vi "Test is a JKI State Machine.vi"(8 "error in (no error)":errorcluster) -> (0 "error out":errorcluster)   [LabVIEW 2013, in "TEST JKI State Machine API.lvlib"]
uses:
  TEST JKI State Machine API.lvlib
  <vilib>/addons/_JKI Toolkits/Caraya/classes/Test/Test.lvclass
  source/JKI SM/JKI SM.lvclass
  <vilib>/addons/_JKI Toolkits/Caraya/classes/Assert/Assert.lvclass
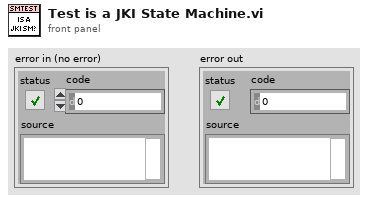
[diagram p1: front panel]
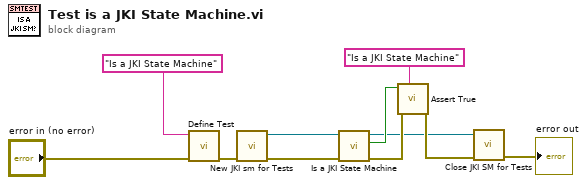
[diagram p0: block diagram]
diagram:
  n1 = call <vilib>:"Define Test.vi"("error in (no error)"="error in (no error)", "Label (VI Title)"="Is a JKI State Machine") -> ("error out"=w7:errorcluster)  [unwired: 9 in]
  n2 = call "New JKI sm for Tests.vi"("error in (no error)"=w7) -> ("error out"=w6:errorcluster, "JKI SM out"=w5:refnum<class "JKI SM.lvclass">)  [unwired: 9 in]
  n3 = call "Is a JKI State Machine.vi"("error in (no error)"=w6, "JKI SM in"=w5) -> ("error out"=w9:errorcluster, "Is a JKI State Machine"=w8:bool, "JKI SM out"=w1:refnum<class "JKI SM.lvclass">)  [unwired: 7 in]
  n4 = call <vilib>:"Assert True.vi"("Label"="Is a JKI State Machine", "error in (no error)"=w9, "True?"=w8) -> ("error out"=w2:errorcluster)  [unwired: 8 in]
  n5 = call "Close JKI SM for Tests.vi"("error in (no error)"=w2, "JKI SM in"=w1) -> ("error out"=→"error out":errorcluster)  [unwired: 9 in]
